vi "set_function.vi"(8 "error in (no error)":errorcluster, 10 "function (0:Sine)":u16(ring) items=["Sine", "Square", "Sine+Noise", "Random", "Chirp"], 11 "NInstrSim_ConfigureWaveformType":refnum<class "NInstrSim_ConfigureWaveformType.lvclass">) -> (0 "error out":errorcluster, 3 "dup NInstrSim_ConfigureWaveformType":refnum<class "NInstrSim_ConfigureWaveformType.lvclass">)   [LabVIEW 2009, in "HB_Device_Examples.lvlib" / "NInstrSim_ConfigureWaveformType.lvclass"]
doc: "Set waveform type"
uses:
  NInstrSim_ConfigureWaveformType.lvclass
  NInstrSim_ConfigureWaveformType.lvclass/NInstrSim_ConfigureWaveformType.ctl
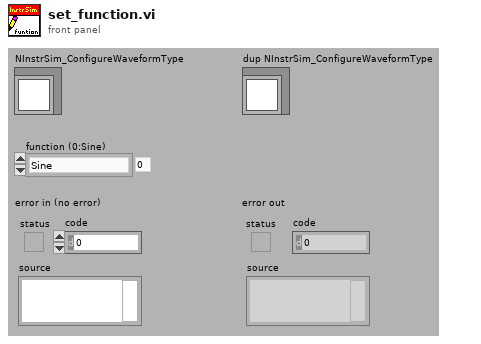
[diagram p1: front panel]
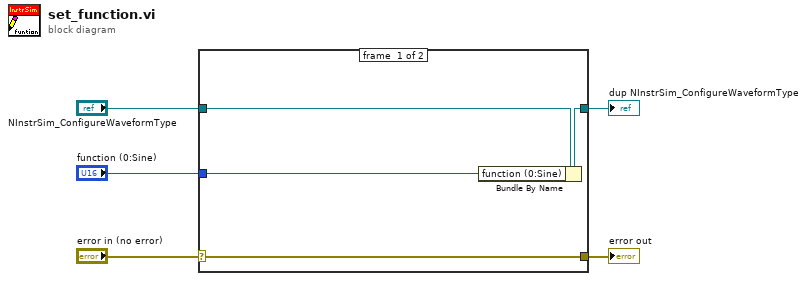
[diagram p0: block diagram]
diagram:
  n1 = case shown="No Error" "error in (no error)" {
    selector: "error in (no error)" -> [w9 w10]
    tunnel: [w9 w10] -> w4
    tunnel: [w7 w11] -> w2
    tunnel: "NInstrSim_ConfigureWaveformType" -> [w8 w11]
    tunnel: "function (0:Sine)" -> [w6 _]
    frame #0 {
      n2 = Bundle By Name(cluster=w8, "function (0:Sine)"=w6) -> (w7:refnum<class "NInstrSim_ConfigureWaveformType.lvclass">)
    }
    frame #1 {
    }
  }
  "error out" <- w4
  "dup NInstrSim_ConfigureWaveformType" <- w2
